vi "Start HD Recorder.vi"(8 "error in (no error)":errorcluster, 9 "Frames":i32, 10 "File":path, 11 "Orca-Flash 4.0 V2 in":refnum<class "Orca-Flash 4.0 V2.lvclass">) -> (0 "error out":errorcluster, 3 "Orca-Flash 4.0 V2 out":refnum<class "Orca-Flash 4.0 V2.lvclass">)   [LabVIEW 2015, in "Orca-Flash 4.0 V2.lvlib" / "Orca-Flash 4.0 V2.lvclass"]
uses:
  Orca-Flash 4.0 V2.lvclass
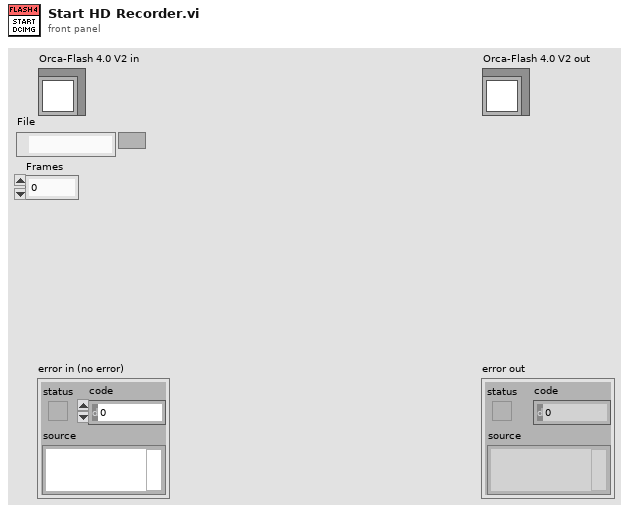
[diagram p1: front panel]
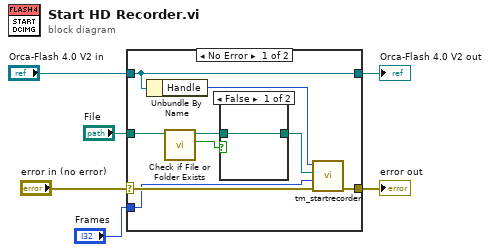
[diagram p0: block diagram]
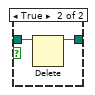
[diagram p2: hidden frame]
diagram:
  n1 = case shown="No Error" "error in (no error)" {
    selector: "error in (no error)" -> [w14 w20]
    tunnel: [w11 w20] -> w5
    tunnel: [w15 w19] -> w3
    tunnel: "Orca-Flash 4.0 V2 in" -> [w15 w19]
    tunnel: "File" -> [w10 _]
    tunnel: "Frames" -> [w12 _]
    frame No Error {
      n2 = Unbundle By Name(w15) -> ("Handle"=w13:u32)
      n3 = call <vilib>:"Check if File or Folder Exists.vi"("path"=w10) -> ("file or folder exists?"=w9:bool, "dup path"=w8:path)  [unwired: 8 in, 1 out]
      n4 = case shown="False" w9 {
        tunnel: w8 -> [w16 w18]
        tunnel: [w16 w17] -> w7
        frame False {
        }
        frame True {
          n5 = Delete(path (use dialog)=w18) -> (deleted path=w17:path)  [unwired: 4 in, 2 out]
        }
      }
      n6 = call <userlib>:"tm_startrecorder.vi"("error in (no error)"=w14, "frames"=w12, "File"=w7, "Handle in"=w13) -> ("error out"=w11:errorcluster)  [unwired: 6 in, 1 out]
    }
    frame Error {
    }
  }
  "error out" <- w5
  "Orca-Flash 4.0 V2 out" <- w3
